vi "CreateModuleRequests.vi"(8 "error in (no error)":errorcluster) -> (0 "error out":errorcluster, 3 "Requests":T1)   [LabVIEW 2024, in "TesterModule.lvclass"]
uses:
  TesterModule.lvclass
  TesterModule.lvclass/TesterModule.ctl
  Request Events--cluster.ctl
  NewControl78732508.ctl
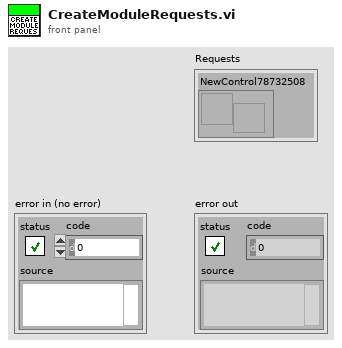
[diagram p1: front panel]
types:
  T1 = typedef "TesterModule.lvclass/Request Events--cluster.ctl" = cluster{"NewControl78732508":refnum<user-event>}
  T2 = typedef "NewControl78732508.ctl" = cluster{"asdf":dbl, "String":string}
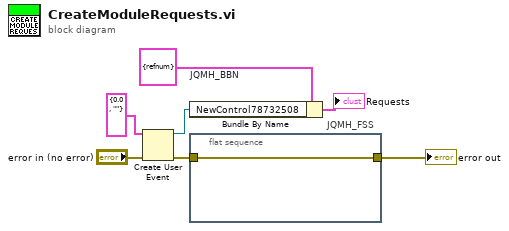
[diagram p0: block diagram]
diagram:
  n1 = Create User Event(user event datatype=T2 {"asdf"=0.0, "String"=""} ("NewControl78732508"), error in="error in (no error)") -> (user event=w3:refnum<user-event>, error out=w1:errorcluster)
  n2 = Bundle By Name "JQMH_BBN"(cluster=T1 {"NewControl78732508"=refnum} ("Requests"), "NewControl78732508"=w3) -> (→"Requests":T1)
  n3 = flat-sequence "JQMH_FSS" {
    tunnel: w1 -> [w8]
    tunnel: [w8] -> w7
    frame #0 {
    }
  }
  "error out" <- w7
